vi "PositionToReceivePassTactic.vi"(5 "Striker/2ndStriker":T1, 6 "Reset":bool, 7 "first call":bool, 8 "error in (no error)":errorcluster, 9 "Robot":refnum<class "Robot.lvclass">, 10 "Game in":refnum<class "Game.lvclass">, 11 "PositionToReceivePassTactic in":refnum<class "PositionToReceivePassTactic.lvclass">) -> (0 "error out":errorcluster, 1 "Sucsses":bool, 2 "Robot out":refnum<class "Robot.lvclass">, 3 "PositionToReceivePassTactic out":refnum<class "PositionToReceivePassTactic.lvclass">)   [LabVIEW 2018, in "PositionToReceivePassTactic.lvclass"]
uses:
  PositionToReceivePassTactic.lvclass
  Robot_class/Robot.lvclass
  Game_class/Game.lvclass
  PreparePassReceiverRole_class/PreparePassReceiverEnum.ctl
  Tactic_class/Tactic.lvclass/Tactic.ctl
  Robot_class/tactics.ctl
  Skillbook_class/Skillbook.lvclass/Skillbook.ctl
  Object_class/Object.lvclass/Object.ctl
  Robot_class/Robot.lvclass/Robot.ctl
  PositionToReceivePassTactic.lvclass/PositionToReceivePassTactic.ctl
  <vilib>/Analysis/_algsub.llb/Real Vector Norm.vi
  Skillbook_class/Read PositionToReceivePassSkill.vi
  Object_class/Read x.vi
  Object_class/Read y.vi
  Robot_class/Read orientation.vi
  Robot_class/Read dest_x.vi
  Robot_class/Read dest_y.vi
  Robot_class/Read dest_orientation.vi
  Tactic_class/Read Skillbook.vi
  Write States.vi
  Robot_class/Write tactic.vi
  Skillbook_class/Skillbook.lvclass
  PositionToReceivePassSkill_class/PositionToReceivePassSkill.lvclass
  <vilib>/Analysis/NI_AALPro.lvlib
panel:
  in  "States in":enum16{"ReceivePass", "Exit"}(ring)
  out "x .or. y?":bool
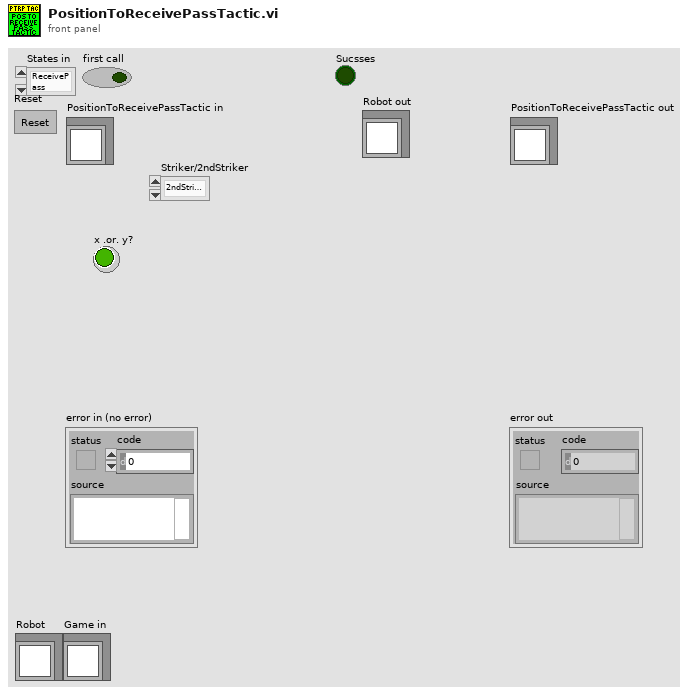
[diagram p1: front panel]
types:
  T1 = typedef "PreparePassReceiverEnum.ctl" = enum16{"2ndStrikerDPass", "2ndStriker", "Striker"}
  T2 = typedef "tactics.ctl" = enum16{"Roller", "PrepareRollToPassRollerGoTo", "PrepareRollToPassReceiverGoTo", "WaitRoll", "PositionToRoll", "PenaltyAttacker", "PassObserver", "PenaltyDefense", "Test", "DefendGoal", "Marker", "FollowAttacker", "DefendArea", "Shoot", "AttackerAimGoal", "AttackerBallOutOfField", "AttackerBlock", "AttackerStop", "Duelist", "Halt", "ZigZag", "GoTo", "Timeout", "KickToPassReceiver", "PositionToReceivePass", "PassReceiver", "WaitPass"}
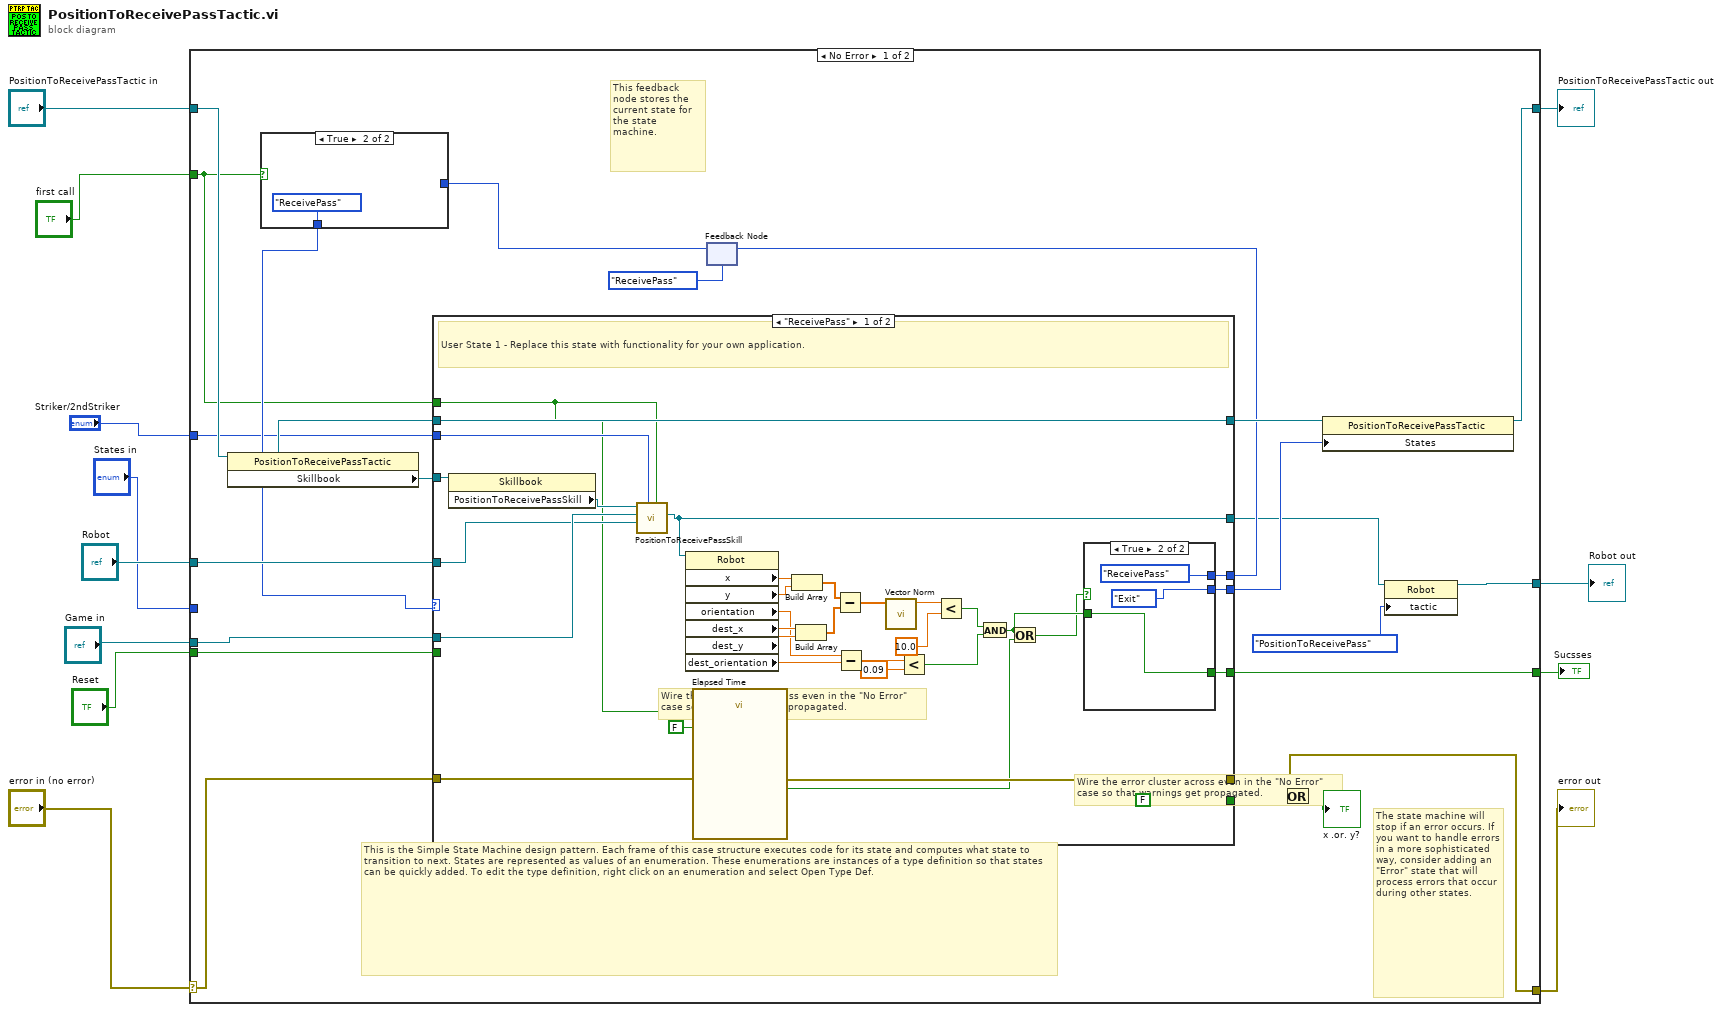
[diagram p0: block diagram]
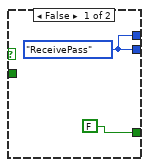
[diagram p3: hidden frame]
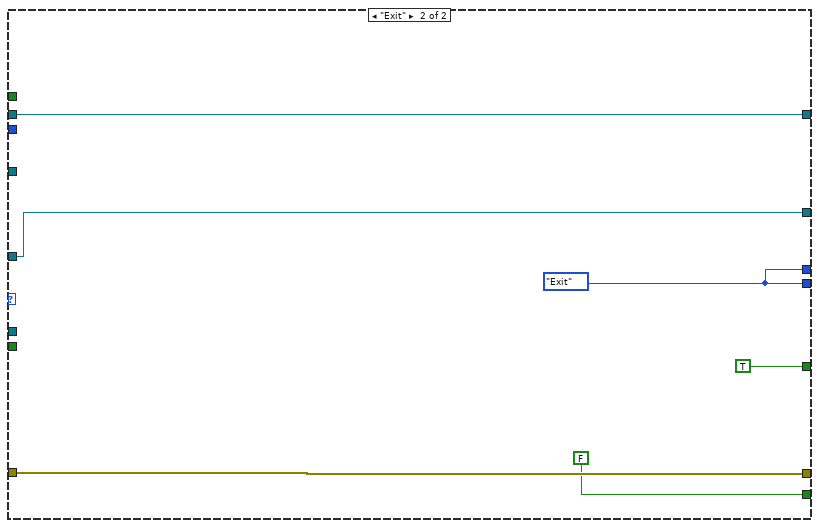
[diagram p4: hidden frame]
diagram:
  n1 = case shown="No Error" "error in (no error)" {
    selector: "error in (no error)" -> [w28 w82]
    tunnel: [w27 w82] -> w11
    tunnel: [w25 w81] -> w9
    tunnel: "PositionToReceivePassTactic in" -> [w26 w81]
    tunnel: "Robot" -> [w30 w80]
    tunnel: "Game in" -> [w29 _]
    tunnel: [w16 w80] -> w6
    tunnel: "States in" -> [_ _]
    tunnel: "Reset" -> [w22 _]
    tunnel: "first call" -> [w14 _]
    tunnel: "Striker/2ndStriker" -> [w15 _]
    tunnel: [w13 _] -> w2
    frame No Error {
      # "The state machine will stop if an error occurs. If you want to handle errors in a more sophisticated way, consider adding an \"Error\" state that will process errors that occur during other states."
      # "This feedback node stores the current state for the state machine."
      # "This is the Simple State Machine design pattern. Each frame of this case structure executes code for its state and computes what state to transition to next. States are represented as values of an enumeration. These enumerations are instances of a type definition so that states can be quickly added. To edit the type definition, right click on an enumeration and select Open Type Def."
      # "Wire the error cluster across even in the \"No Error\"\ncase so that warnings get propagated."
      # "Wire the error cluster across even in the \"No Error\"\ncase so that warnings get propagated."
      n2 = property class="PositionToReceivePassTactic"(reference=w26) -> ("Skillbook"=w32:refnum<class "Skillbook.lvclass">)  [unwired: 1 in, 2 out]
      n3 = feedback #1(enum16{"ReceivePass", "Exit"}."ReceivePass" ("States")) -> (w19:enum16{"ReceivePass", "Exit"})
      n4 = case shown="True" w14 {
        tunnel: [w35 enum16{"ReceivePass", "Exit"}."ReceivePass" ("States")] -> w20
        tunnel: w19 -> [w35 _]
        frame False {
        }
        frame True {
        }
      }
      n5 = case shown="\"ReceivePass\"" w20 {
        tunnel: [FALSE ("Stop Loop?") FALSE ("Stop Loop?")] -> w34
        tunnel: w32 -> [w67 _]
        tunnel: w30 -> [w62 w78]
        tunnel: [w60 w78] -> w17
        tunnel: [w66 w79] -> w31
        tunnel: w26 -> [w66 w79]
        tunnel: w29 -> [w64 _]
        tunnel: [w63 w77] -> w27
        tunnel: w28 -> [w63 w77]
        tunnel: [w61 w75] -> w24
        tunnel: w22 -> [_ _]
        tunnel: [w44 w75] -> w21
        tunnel: w15 -> [w43 _]
        tunnel: w14 -> [w41 _]
        tunnel: [w39 TRUE] -> w13
        frame "ReceivePass" {
          # "User State 1 - Replace this state with functionality for your own application."
          n6 = property class="Skillbook"(reference=w67) -> ("PositionToReceivePassSkill"=w65:refnum<class "PositionToReceivePassSkill.lvclass">)  [unwired: 1 in, 2 out]
          n7 = call "PositionToReceivePassSkill.vi"("first call"=w41, "Striker/2ndStriker"=w43, "Robot"=w62, "Game"=w64, "PositionToReceivePassSkill in"=w65) -> ("Robot out"=w60:refnum<class "Robot.lvclass">)  [unwired: 4 in, 2 out]
          n8 = property class="Robot"(reference=w60) -> ("x"=w59:dbl, "y"=w58:dbl, "orientation"=w53:dbl, "dest_x"=w57:dbl, "dest_y"=w56:dbl, "dest_orientation"=w52:dbl)  [unwired: 1 in, 2 out]
          n9 = call "Elapsed Time"("Reset"=w41, "Auto Reset"=FALSE) -> ("Time has Elapsed"=w42:bool)  [unwired: 10 in, 7 out]
          n10 = Build Array(w59, w58) -> (w55:dbl[])
          n11 = Build Array(w57, w56) -> (w54:dbl[])
          n12 = Subtract(x=w55, y=w54) -> (x-y=w51:dbl[])
          n13 = Subtract(x=w53, y=w52) -> (x-y=w48:dbl)
          n14 = call-poly <vilib>:"Vector Norm.vi"("Input Vector"=w51) -> ("norm"=w50:dbl)  [unwired: 9 in, 1 out]
          n15 = Less?(x=w48, y=0.09) -> (x < y?=w45:bool)
          n16 = Less?(x=w50, y=10.0) -> (x < y?=w46:bool)
          n17 = And(x=w46, y=w45) -> (x .and. y?=w38:bool)
          n18 = Or(x=w38, y=w42) -> (x .or. y?=w37:bool)
          n19 = case shown="True" w37 {
            tunnel: [w70 enum16{"ReceivePass", "Exit"}."Exit" ("States")] -> w61
            tunnel: [w70 enum16{"ReceivePass", "Exit"}."ReceivePass" ("States")] -> w44
            tunnel: [FALSE w71] -> w39
            tunnel: w38 -> [_ w71]
            frame False {
              w70 = enum16{"ReceivePass", "Exit"}."ReceivePass" ("States")
            }
            frame True {
            }
          }
        }
        frame "Exit" {
          w75 = enum16{"ReceivePass", "Exit"}."Exit" ("States")
        }
      }
      n20 = feedback-in #1(w21) -> ()
      n21 = Or(x=w27, y=w34) -> (x .or. y?=→"x .or. y?":bool)
      n22 = property class="PositionToReceivePassTactic"(reference=w31, "States"=w24) -> (reference out=w25:refnum<class "PositionToReceivePassTactic.lvclass">)  [unwired: 1 in, 1 out]
      n23 = property class="Robot"(reference=w17, "tactic"=tactics."PositionToReceivePass") -> (reference out=w16:refnum<class "Robot.lvclass">)  [unwired: 1 in, 1 out]
    }
    frame Error {
    }
  }
  "error out" <- w11
  "PositionToReceivePassTactic out" <- w9
  "Robot out" <- w6
  "Sucsses" <- w2
